vi "OpenDeviceByIndex.vi"(0 "nDeviceIndex":u32, 1 "error in (no error)":errorcluster) -> (2 "phDevice":u64, 3 "GX_STATUS":i32, 4 "error out":errorcluster)   [LabVIEW 2016, in "GxLVLib.lvlib"]
uses:
  GxLVLib.lvlib
  GxIAPI.dll
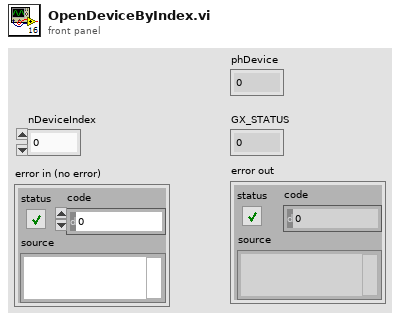
[diagram p1: front panel]
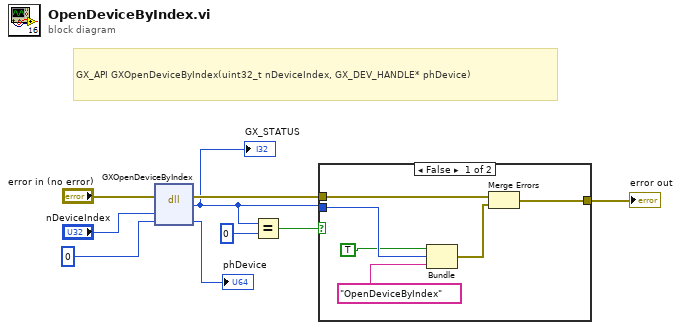
[diagram p0: block diagram]
diagram:
  # "GX_API GXOpenDeviceByIndex(uint32_t nDeviceIndex, GX_DEV_HANDLE* phDevice)"
  n1 = dll-call lib="GxIAPI.dll" fn="GXOpenDeviceByIndex"(error in="error in (no error)", "nDeviceIndex"="nDeviceIndex", "phDevice"=u64 0) -> (error out=w5:errorcluster, "GX_STATUS"=w1:i32, "phDevice"=→"phDevice":i64)  [unwired: 3 in, 1 out]
  "GX_STATUS" <- w1
  n2 = Equal?(x=w1, y=0) -> (x = y?=w3:bool)
  n3 = case shown="False" w3 {
    tunnel: w5 -> [w15 w16]
    tunnel: [w14 w16] -> w6
    tunnel: w1 -> [w11 _]
    frame False {
      n4 = Bundle(TRUE, "GX_STATUS"=w11, "OpenDeviceByIndex") -> (w12:cluster{bool, "GX_STATUS":i32, string})  [unwired: 1 in]
      n5 = Merge Errors(w15, w12) -> (w14:errorcluster)
    }
    frame True {
    }
  }
  "error out" <- w6
